vi "modbus initialize API object.vi"(8 "error in":errorcluster, 11 "Modbus Slave configuration in":refnum<class "Modbus Module configuration.lvclass">) -> (0 "error out":errorcluster, 3 "Modbus Slave out":refnum<class "Modbus API.lvclass">)   [LabVIEW 2014, in "Modbus Module runtime.lvclass"]
uses:
  Modbus Module runtime.lvclass
  configuration/Modbus Module configuration.lvclass
  <vilib>/NI/Modbus Library/API/Modbus API.lvclass
  configuration/Modbus Module configuration.lvclass/Modbus Module configuration.ctl
  <vilib>/NI/Modbus Library/API/Master/Modbus Master.lvclass
  configuration/Read port (502).vi
  configuration/Read IP address.vi
  configuration/Read serial type.vi
  configuration/Read unit ID.vi
  configuration/Read VISA resource name.vi
  configuration/Read baud rate.vi
  configuration/Read parity (even).vi
  configuration/Read flow control (none).vi
  configuration/Read class.vi
  <vilib>/NI/Modbus Library/API/Wrapper/Create TCP Slave.vi
  <vilib>/NI/Modbus Library/API/Wrapper/Create TCP Master.vi
  configuration/read force wire mode.vi
  configuration/get wire mode.vi
  <vilib>/NI/Modbus Library/API/Wrapper/Create Serial Master.vi
  <vilib>/NI/Modbus Library/API/Wrapper/Create Serial Slave.vi
  <vilib>/NI/Modbus Library/API/Wrapper/API Main.lvlib
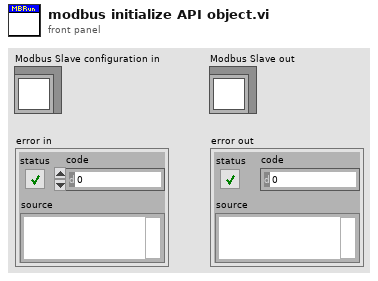
[diagram p1: front panel]
types:
  T1 = typedef "Modbus Slave configuration.lvclass/modbus class.ctl" = enum16{"TCP master", "TCP slave", "serial master", "serial slave"}
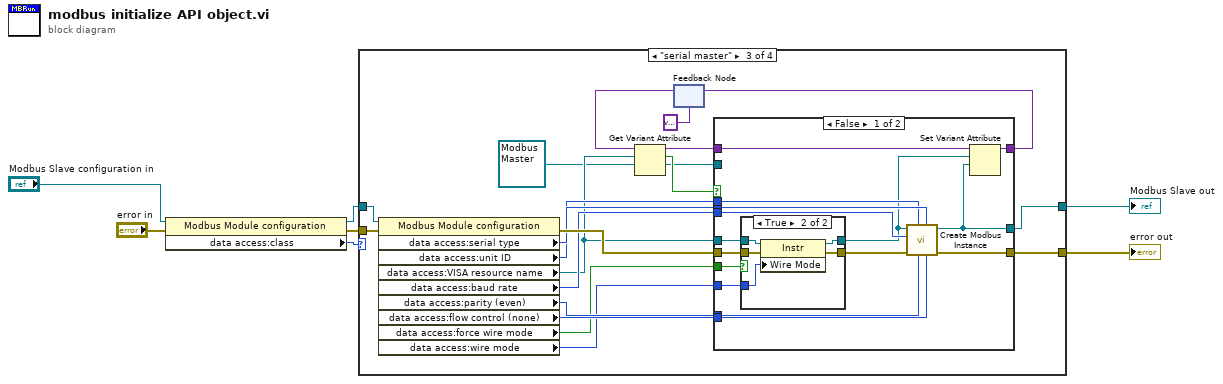
[diagram p0: block diagram]
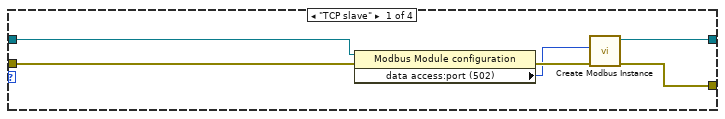
[diagram p2: hidden frame]
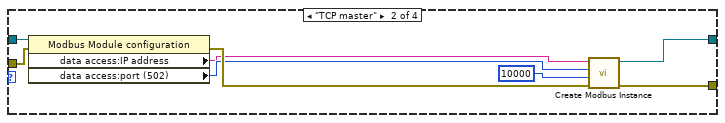
[diagram p3: hidden frame]
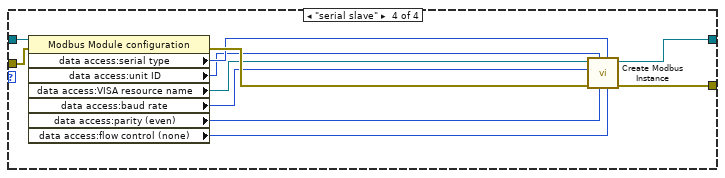
[diagram p6: hidden frame]
diagram:
  n1 = property class="Modbus Module configuration"(reference="Modbus Slave configuration in", error in="error in") -> (reference out=w1:refnum<class "Modbus Module configuration.lvclass">, error out=w4:errorcluster, "data access:class"=w2:T1)
  n2 = case shown="\"serial master\"" w2 {
    tunnel: [w13 w21 w41 w77] -> w7
    tunnel: [w12 w20 w40 w76] -> w5
    tunnel: w4 -> [w11 w19 w39 w75]
    tunnel: w1 -> [w9 w17 w37 w73]
    frame "TCP slave" {
      n3 = property class="Modbus Module configuration"(reference=w9, error in=w11) -> (error out=w10:errorcluster, "data access:port (502)"=w8:u16)  [unwired: 1 out]
      n4 = call-poly <vilib>:"Create Modbus Instance.vi"("error in"=w10, "port (502)"=w8) -> ("error out"=w13:errorcluster, "TCP slave instance"=w12:refnum<class "Modbus Slave.lvclass">)  [unwired: 8 in]
    }
    frame "TCP master" {
      n5 = property class="Modbus Module configuration"(reference=w17, error in=w19) -> (error out=w18:errorcluster, "data access:IP address"=w14:string, "data access:port (502)"=w16:u16)  [unwired: 1 out]
      n6 = call-poly <vilib>:"Create Modbus Instance.vi"("error in"=w18, "connect timeout ms"=10000, "port (502)"=w16, "address"=w14) -> ("error out"=w21:errorcluster, "TCP master instance"=w20:refnum<class "Modbus Master.lvclass">)  [unwired: 6 in]
    }
    frame "serial master" {
      n7 = property class="Modbus Module configuration"(reference=w37, error in=w39) -> (error out=w38:errorcluster, "data access:serial type"=w36:enum16{"RTU", "ASCII"}, "data access:unit ID"=w35:u8, "data access:VISA resource name"=w27:refnum<visa-resource-name>, "data access:baud rate"=w34:u32, "data access:parity (even)"=w33:u16, "data access:flow control (none)"=w32:u16, "data access:force wire mode"=w31:bool, "data access:wire mode"=w30:i16)  [unwired: 1 out]
      n8 = feedback #1(variant) -> (w28:variant)
      n9 = Get Variant Attribute(Variant=w28, name=w27, default value (empty Variant)=refnum<class "Modbus Master.lvclass"> refnum ("serial master instance")) -> (duplicate Variant=w24:variant, found=w25:bool, value=w23:refnum<class "Modbus Master.lvclass">)  [unwired: 1 in, 1 out]
      n10 = case shown="False" w25 {
        tunnel: [w56 w65] -> w41
        tunnel: [w44 w66] -> w40
        tunnel: w38 -> [w55 w65]
        tunnel: w36 -> [w54 _]
        tunnel: w35 -> [w53 _]
        tunnel: w34 -> [w52 _]
        tunnel: w33 -> [w51 _]
        tunnel: w32 -> [w50 _]
        tunnel: w31 -> [w48 _]
        tunnel: w30 -> [w47 _]
        tunnel: w27 -> [w46 _]
        tunnel: w24 -> [w45 w64]
        tunnel: w23 -> [_ w66]
        tunnel: [w42 w64] -> w22
        frame False {
          n11 = case shown="True" w48 {
            tunnel: w55 -> [w57 w63]
            tunnel: [w57 w62] -> w49
            tunnel: w46 -> [w58 w61]
            tunnel: [w58 w60] -> w43
            tunnel: w47 -> [_ w59]
            frame False {
            }
            frame True {
              n12 = property class="Instr"(reference=w61, error in=w63, "Wire Mode"=w59) -> (reference out=w60:refnum<visa-resource-name>, error out=w62:errorcluster)
            }
          }
          n13 = call-poly <vilib>:"Create Modbus Instance.vi"("flow control (none)"=w50, "serial type"=w54, "parity (even)"=w51, "unit ID"=w53, "error in"=w49, "baud rate"=w52, "VISA resource name"=w43) -> ("error out"=w56:errorcluster, "serial master instance"=w44:refnum<class "Modbus Master.lvclass">)  [unwired: 3 in]
          n14 = Set Variant Attribute(Variant=w45, name=w43, value=w44) -> (Variant out=w42:variant)  [unwired: 1 in, 2 out]
        }
        frame True {
        }
      }
      n15 = feedback-in #1(w22) -> ()
    }
    frame "serial slave" {
      n16 = property class="Modbus Module configuration"(reference=w73, error in=w75) -> (error out=w74:errorcluster, "data access:serial type"=w72:enum16{"RTU", "ASCII"}, "data access:unit ID"=w71:u8, "data access:VISA resource name"=w70:refnum<visa-resource-name>, "data access:baud rate"=w69:u32, "data access:parity (even)"=w68:u16, "data access:flow control (none)"=w67:u16)  [unwired: 1 out]
      n17 = call-poly <vilib>:"Create Modbus Instance.vi"("flow control"=w67, "serial type"=w72, "parity (even)"=w68, "unit ID"=w71, "error in"=w74, "baud rate (9600)"=w69, "VISA resource name"=w70) -> ("error out"=w77:errorcluster, "serial slave instance"=w76:refnum<class "Modbus Slave.lvclass">)  [unwired: 3 in]
    }
  }
  "error out" <- w7
  "Modbus Slave out" <- w5
